vi "Get Table.vi"(7 "Name":string, 8 "error in (no error)":errorcluster, 11 "Form Server Wrapper in":refnum<class "Form Server Wrapper.lvclass">) -> (0 "error out":errorcluster, 2 "Table":refnum<class "Basic Table.lvclass">, 3 "Form Server Wrapper out":refnum<class "Form Server Wrapper.lvclass">)   [LabVIEW 2020, in "Form Server.lvlib" / "Form Server Wrapper.lvclass"]
uses:
  Form Server Wrapper.lvclass
  Database OOP/Table Libraries/Basic Table/Basic Table Class/Basic Table.lvclass
  Form Server Wrapper.lvclass/Form Server Wrapper.ctl
  Form Server Messages Messages/Get Table Object Msg/Get Table Object Msg.lvclass/Get Table Object Msg.ctl
  <vilib>/ActorFramework/Reply Msg/Reply Msg.lvclass/Reply Msg.ctl
  <vilib>/ActorFramework/Message Enqueuer/Message Enqueuer.lvclass/Message Enqueuer.ctl
  <vilib>/ActorFramework/Reply Msg/Send Message And Wait For Response.vi
  <vilib>/ActorFramework/Message Enqueuer/Enqueue.vi
  Form Server Messages Messages/Get Table Object Msg/Get Table Object Msg.lvclass
  C:/Program Files (x86)/National Instruments/LabVIEW 2020/vi.lib/ActorFramework/Reply Msg/Reply Msg.lvclass
  <vilib>/ActorFramework/Reply Msg/Reply Msg.lvclass
  C:/Program Files (x86)/National Instruments/LabVIEW 2020/vi.lib/ActorFramework/Message/Message.lvclass
  <vilib>/ActorFramework/Message Priority Queue/Priority Enqueue.vi
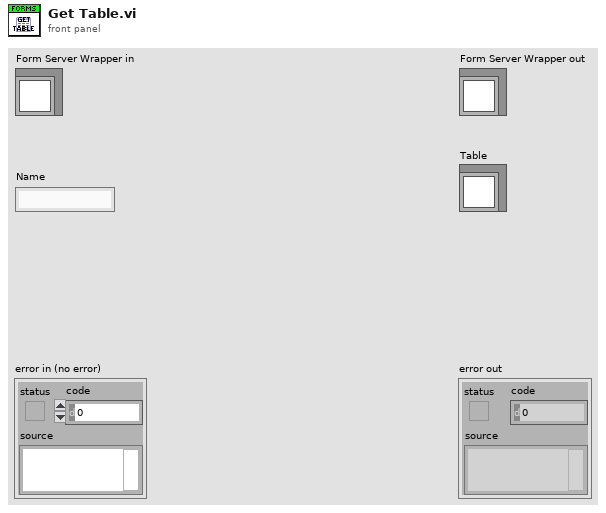
[diagram p1: front panel]
types:
  T1 = typedef "Form Server Interfaces.lvlib/Form ID.ctl" = cluster{"Name":string, "Panel type":string}
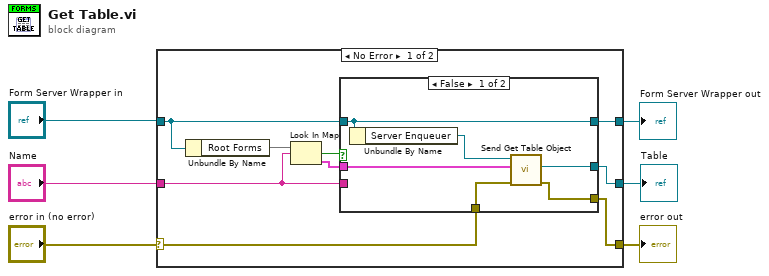
[diagram p0: block diagram]
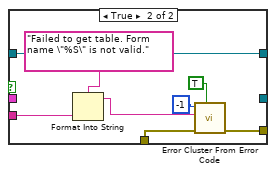
[diagram p2: hidden frame]
diagram:
  n1 = case shown="No Error" "error in (no error)" {
    selector: "error in (no error)" -> [w14 w31]
    tunnel: [w13 w31] -> w3
    tunnel: [w15 w30] -> w5
    tunnel: "Form Server Wrapper in" -> [w12 w30]
    tunnel: "Name" -> [w8 _]
    tunnel: [w7 _] -> w1
    frame No Error {
      n2 = Unbundle By Name(w12) -> ("Root Forms"=w11:map{string, T1})
      n3 = Look In Map(map=w11, key=w8) -> (key not found?=w10:bool, value=w9:T1)  [unwired: 1 in]
      n4 = case shown="False" w10 {
        tunnel: w9 -> [w19 _]
        tunnel: w12 -> [w21 w26]
        tunnel: [w21 w26] -> w15
        tunnel: w14 -> [w18 w29]
        tunnel: w8 -> [_ w24]
        tunnel: [w17 w22] -> w13
        tunnel: [w16 _] -> w7
        frame False {
          n5 = Unbundle By Name(w21) -> ("Server Enqueuer"=w20:refnum<class "Message Enqueuer.lvclass">)
          n6 = call "Send Get Table Object.vi"("error in (no error)"=w18, "Form ID"=w19, "Message Enqueuer"=w20) -> ("error out"=w17:errorcluster, "Table"=w16:refnum<class "Basic Table.lvclass">)  [unwired: 5 in, 2 out]
        }
        frame True {
          n7 = Format Into String(format string="Failed to get table. Form name \"%S\" is not valid.", w24) -> (resulting string=w23:string)  [unwired: 2 in, 1 out]
          n8 = call <vilib>:"Error Cluster From Error Code.vi"("show call chain? (False)"=TRUE, "error in (no error)"=w29, "error message (\"\")"=w23, "error code (0)"=-1) -> ("error out"=w22:errorcluster)  [unwired: 5 in]
        }
      }
    }
    frame Error {
    }
  }
  "error out" <- w3
  "Form Server Wrapper out" <- w5
  "Table" <- w1
